vi "Message Is Valid.vi"(11 "Message":u8[](array[numeric]) format="%.0x") -> (3 "Valid":bool)   [LabVIEW 2015, in "VC940.lvlib"]
uses:
  VC940.lvlib
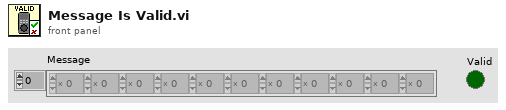
[diagram p1: front panel]
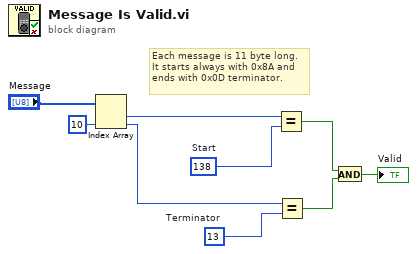
[diagram p0: block diagram]
diagram:
  w5 = u8 13  # Terminator
  w6 = u8 138  # Start
  # "Each message is 11 byte long.\nIt starts always with 0x8A and\nends with 0x0D terminator."
  n1 = Index Array(array="Message", index #2=10 ("index")) -> (element #1=w8:u8, element #2=w7:u8)  [unwired: 1 in]
  n2 = Equal?(x=w8, y=w6) -> (x = y?=w4:bool)
  n3 = Equal?(x=w7, y=w5) -> (x = y?=w3:bool)
  n4 = And(x=w4, y=w3) -> (x .and. y?=→"Valid":bool)
